vi "Maquina01Refrescos.vi"() -> ()   [LabVIEW 2018]
uses:
  EdoMaq1Refrescos.ctl
panel:
  out "Elapsed Time (s)":dbl
  out "Cambio":i32
  out "Suma":i32
  out "Edo":T1
  in  "stop":bool
  in  "Cancel Button":bool
  in  "$10":bool
  in  "$5":bool
  in  "$1":bool
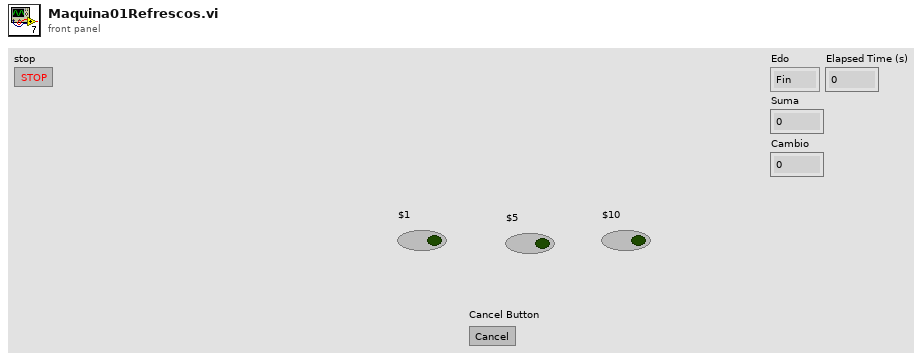
[diagram p1: front panel]
types:
  T1 = typedef "EdoMaq1Refrescos.ctl" = enum16{"Fin", "Espera", "JuntaDinero", "Entrega", "RegresaCambio", "Cancela"}
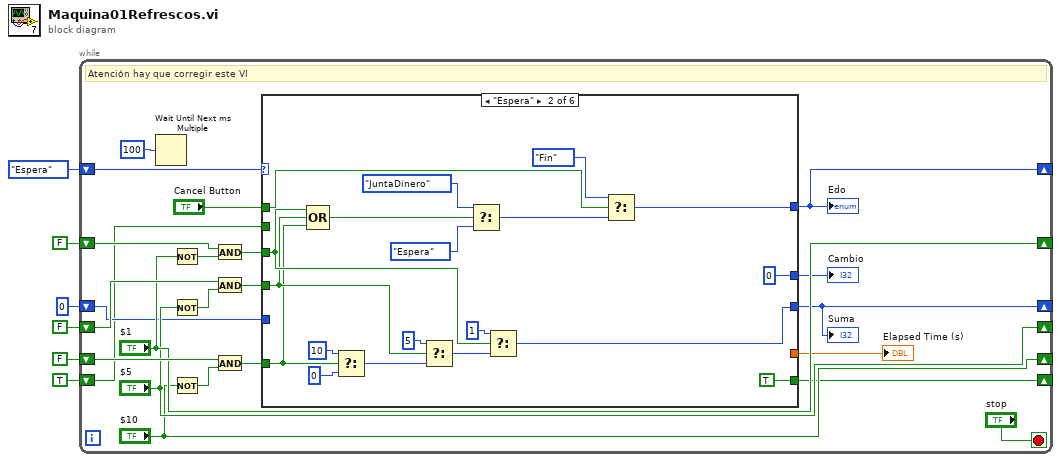
[diagram p0: block diagram]
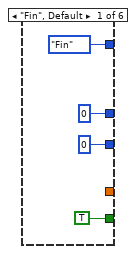
[diagram p2: hidden frame]
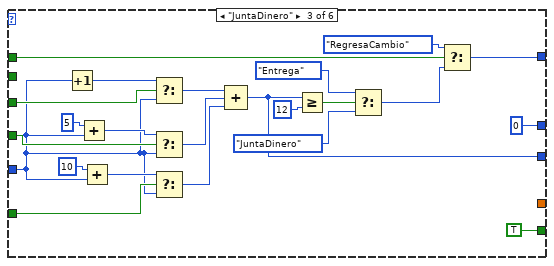
[diagram p3: hidden frame]
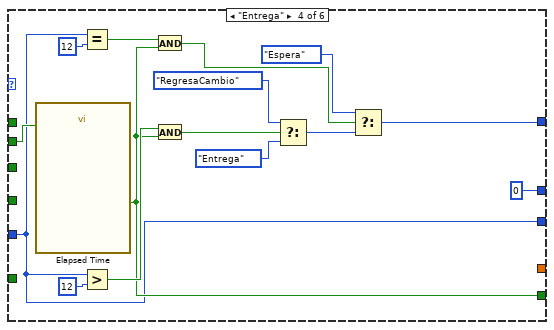
[diagram p4: hidden frame]
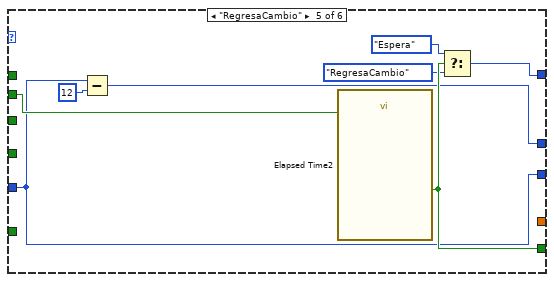
[diagram p5: hidden frame]
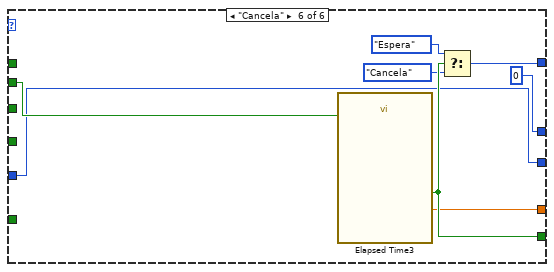
[diagram p6: hidden frame]
diagram:
  n1 = while {
    shift-right: [w13] -> _
    shift-left: EdoMaq1Refrescos."Espera" -> [w27]
    shift-right: ["$1"] -> _
    shift-left: FALSE -> [w25]
    shift-right: ["$5"] -> _
    shift-left: FALSE -> [w24]
    shift-right: ["$10"] -> _
    shift-left: FALSE -> [w23]
    shift-right: [w11] -> _
    shift-left: 0 -> [w12]
    shift-right: [w9] -> _
    shift-left: TRUE -> [w10]
    stop <- "stop" stop-if-true
    # "Atención hay que corregir este VI"
    n2 = Wait Until Next ms Multiple(millisecond multiple=u32 100) -> ()  [unwired: 1 out]
    n3 = Not(x="$1") -> (.not. x?=w22:bool)
    n4 = Not(x="$5") -> (.not. x?=w21:bool)
    n5 = Not(x="$10") -> (.not. x?=w20:bool)
    n6 = And(x=w25, y=w22) -> (x .and. y?=w19:bool)
    n7 = And(x=w24, y=w21) -> (x .and. y?=w18:bool)
    n8 = And(x=w23, y=w20) -> (x .and. y?=w17:bool)
    n9 = case shown="\"Espera\"" w27 {
      tunnel: "Cancel Button" -> [_ w51 w74 _ _ _]
      tunnel: w19 -> [_ w45 w72 _ _ _]
      tunnel: w18 -> [_ w42 w70 _ _ _]
      tunnel: w17 -> [_ w40 w67 _ _ _]
      tunnel: [EdoMaq1Refrescos."Fin" ("f") w47 w56 w78 w94 w102] -> w13
      tunnel: w12 -> [_ _ w64 w77 w91 w100]
      tunnel: [0 w36 w55 w77 w91 w100] -> w11
      tunnel: w10 -> [_ _ _ w90 w98 w106]
      tunnel: [TRUE ("Time has Elapsed") TRUE ("Time has Elapsed") TRUE ("Time has Elapsed") w82 w97 w105] -> w9
      tunnel: [0 0 0 0 w92 0] -> w8
      tunnel: [_ _ _ _ _ w99] -> w7
      frame "Fin", Default {
      }
      frame "Espera" {
        n10 = Compound Arithmetic op=OR(w45, w42, w40) -> (w48:bool)
        n11 = Select(t=10, s=w40, f=0) -> (s? t:f=w38:i32)
        n12 = Select(t=5, s=w42, f=w38) -> (s? t:f=w43:i32)
        n13 = Select(t=EdoMaq1Refrescos."JuntaDinero", s=w48, f=EdoMaq1Refrescos."Espera") -> (s? t:f=w52:T1)
        n14 = Select(t=1, s=w45, f=w43) -> (s? t:f=w36:i32)
        n15 = Select(t=EdoMaq1Refrescos."Fin", s=w51, f=w52) -> (s? t:f=w47:T1)
      }
      frame "JuntaDinero" {
        n16 = Increment(x=w64) -> (x+1=w71:i32)
        n17 = Add(x=5, y=w64) -> (x+y=w68:i32)
        n18 = Add(x=10, y=w64) -> (x+y=w65:i32)
        n19 = Select(t=w71, s=w72, f=w64) -> (s? t:f=w63:i32)
        n20 = Select(t=w68, s=w70, f=w64) -> (s? t:f=w62:i32)
        n21 = Select(t=w65, s=w67, f=w64) -> (s? t:f=w61:i32)
        n22 = Compound Arithmetic op=ADD(w63, w62, w61) -> (w55:i32)
        n23 = Greater Or Equal?(x=w55, y=12) -> (x >= y?=w59:bool)
        n24 = Select(t=EdoMaq1Refrescos."Entrega", s=w59, f=EdoMaq1Refrescos."JuntaDinero") -> (s? t:f=w75:T1)
        n25 = Select(t=EdoMaq1Refrescos."RegresaCambio", s=w74, f=w75) -> (s? t:f=w56:T1)
      }
      frame "Entrega" {
        n26 = call "Elapsed Time"("Reset"=w90) -> ("Time has Elapsed"=w82:bool)  [unwired: 11 in, 7 out]
        n27 = Equal?(x=w77, y=12) -> (x = y?=w87:bool)
        n28 = Greater?(x=w77, y=12) -> (0:w83:bool)
        n29 = And(x=w87, y=w82) -> (x .and. y?=w86:bool)
        n30 = And(x=w83, y=w82) -> (x .and. y?=w81:bool)
        n31 = Select(t=EdoMaq1Refrescos."RegresaCambio", s=w81, f=EdoMaq1Refrescos."Entrega") -> (s? t:f=w89:T1)
        n32 = Select(t=EdoMaq1Refrescos."Espera", s=w86, f=w89) -> (s? t:f=w78:T1)
      }
      frame "RegresaCambio" {
        n33 = Subtract(x=w91, y=12) -> (x-y=w92:i32)
        n34 = call "Elapsed Time2"("Reset"=w98) -> ("Time has Elapsed"=w97:bool)  [unwired: 11 in, 7 out]
        n35 = Select(t=EdoMaq1Refrescos."Espera", s=w97, f=EdoMaq1Refrescos."RegresaCambio") -> (s? t:f=w94:T1)
      }
      frame "Cancela" {
        n36 = call "Elapsed Time3"("Reset"=w106) -> ("Elapsed Time (s)"=w99:dbl, "Time has Elapsed"=w105:bool)  [unwired: 11 in, 6 out]
        n37 = Select(t=EdoMaq1Refrescos."Espera", s=w105, f=EdoMaq1Refrescos."Cancela") -> (s? t:f=w102:T1)
      }
    }
    "Edo" <- w13
    "Suma" <- w11
    "Cambio" <- w8
    "Elapsed Time (s)" <- w7
  }
